vi "TCP - Wait.vi"(8 "error in":errorcluster, 11 "TCP Network Connection in":refnum<k5>) -> (0 "error out":errorcluster, 3 "TCP Network Connection out":refnum<k5>)   [LabVIEW 2021]
doc: "Create a delay, to allow the device enough time to receive the command.\n\nThe wait time is defined by the constant VI \"Constant - TCP Wait Time (ms)\"."
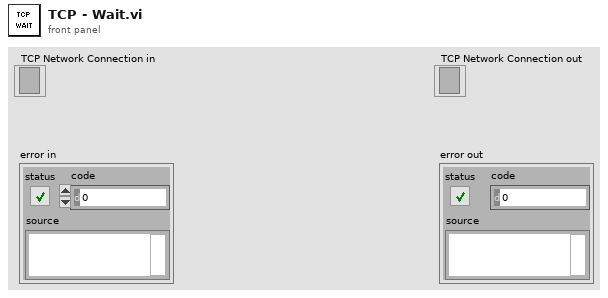
[diagram p1: front panel]
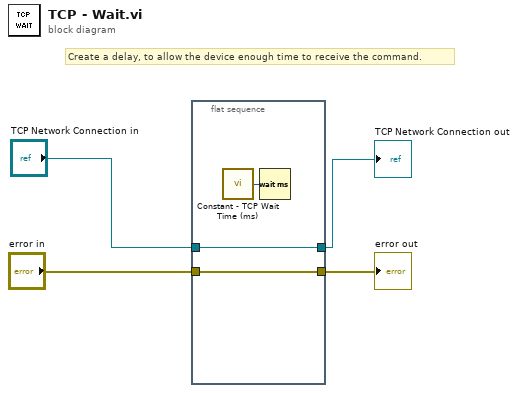
[diagram p0: block diagram]
diagram:
  # "Create a delay, to allow the device enough time to receive the command."
  n1 = flat-sequence {
    tunnel: "error in" -> [w7]
    tunnel: [w7] -> w2
    tunnel: "TCP Network Connection in" -> [w6]
    tunnel: [w6] -> w4
    frame #0 {
      n2 = call "Constant - TCP Wait Time (ms).vi"() -> ("milliseconds to wait"=w5:u32)  [unwired: 11 in]
      n3 = Wait (ms)(milliseconds to wait=w5) -> ()  [unwired: 1 out]
    }
  }
  "TCP Network Connection out" <- w4
  "error out" <- w2
